vi "MRU_UpdateMRUList.vi"(8 "error in (no error)":errorcluster, 11 "reference in":refnum<class "MRU.lvclass">) -> (0 "error out":errorcluster, 3 "reference out":refnum<class "MRU.lvclass">)   [LabVIEW 2014, in "MRU.lvclass"]
doc: "Captures the current values in the Combo Box and saves them to the INI file given to the constructor."
uses:
  MRU.lvclass
  <vilib>/Utility/config.llb/Write Key (String).vi
  <vilib>/Utility/config.llb/NI_LVConfig.lvlib
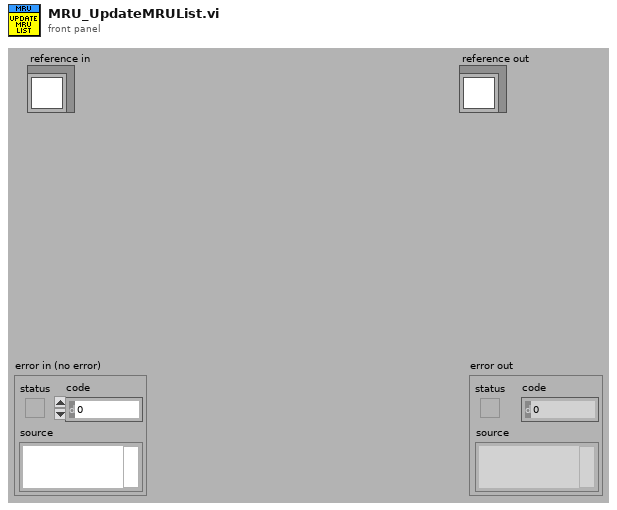
[diagram p1: front panel]
types:
  T1 = typedef "MRU.lvclass/ObjectAttributes.ctl" = cluster{"MRU INI file":path, "MRU Section Name":string, "CmbBox Refnum":refnum<vi>, "Number to remember":i32}
  T2 = typedef "NI_LVConfig.lvlib/Config Data RefNum.ctl" = refnum<k1>
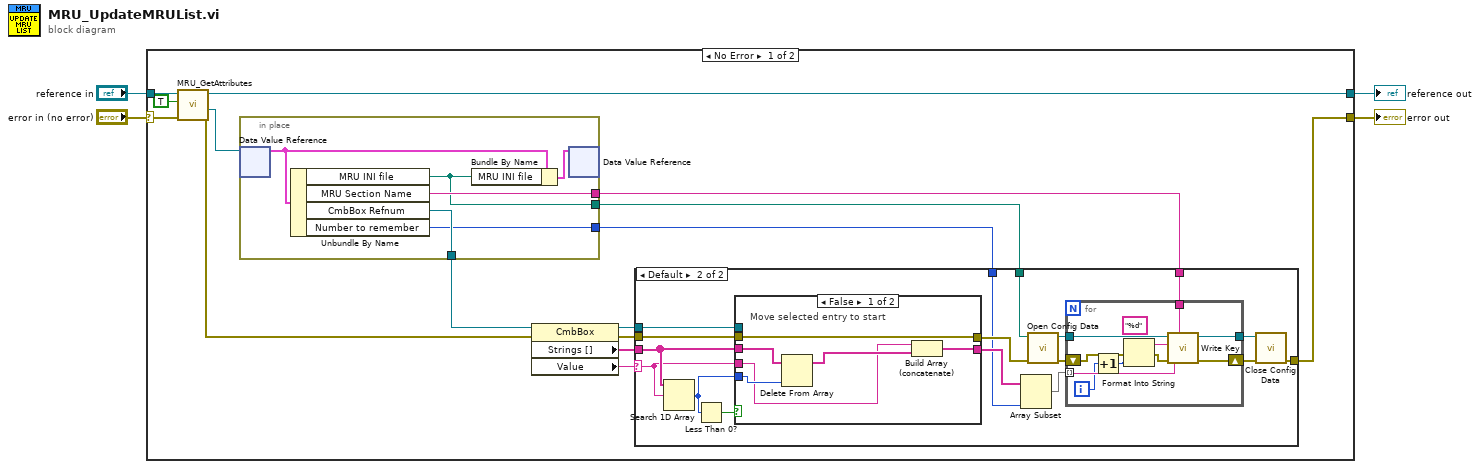
[diagram p0: block diagram]
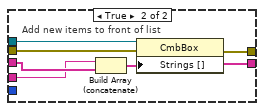
[diagram p3: hidden frame]
diagram:
  n1 = case shown="No Error" "error in (no error)" {
    selector: "error in (no error)" -> [w17 w68]
    tunnel: [w19 w68] -> w3
    tunnel: [w16 w67] -> w1
    tunnel: "reference in" -> [w18 w67]
    frame No Error {
      n2 = call "MRU_GetAttributes.vi"("error in (no error)"=w17, "OnlyGetDvrReference(False)"=TRUE, "reference in"=w18) -> ("error out"=w12:errorcluster, "DataRef"=w10:refnum<data-value>, "reference out"=w16:refnum<class "MRU.lvclass">)  [unwired: 5 in, 1 out]
      n3 = in-place {
        in-place-border: [w64] -> w9
        in-place-border: [w63] -> w8
        in-place-border: [w62] -> w7
        in-place-border: [w61] -> w6
        n4 = in-place-dvr #1(w10) -> (w66:T1)  [unwired: 1 out]
        n5 = Unbundle By Name(w66) -> ("MRU INI file"=w61:path, "MRU Section Name"=w64:string, "CmbBox Refnum"=w63:refnum<vi>, "Number to remember"=w62:i32)
        n6 = Bundle By Name(cluster=w66, "MRU INI file"=w61) -> (w65:T1)
        n7 = in-place-dvr #1(w65) -> ()  [unwired: 2 out]
      }
      n8 = property on="Property Node" class="CmbBox"(reference=w8, error in=w12) -> (reference out=w13:refnum<vi>, error out=w14:errorcluster, "Strings []"=w15:string[], "Value"=w5:string)
      n9 = case shown="Default" w5 {
        selector: w5 -> [_ w21]
        tunnel: [w20 w37] -> w19
        tunnel: w15 -> [_ w35]
        tunnel: w14 -> [w20 w34]
        tunnel: w13 -> [_ w28]
        tunnel: w9 -> [_ w24]
        tunnel: w7 -> [_ w23]
        tunnel: w6 -> [_ w22]
        frame "\u0000" {
        }
        frame Default {
          n10 = Search 1D Array(1D array=w35, element=w21) -> (index of element=w25:i32)  [unwired: 1 out]
          n11 = Less Than 0?(x=w25) -> (x < 0?=w36:bool)
          n12 = case shown="False" w36 {
            tunnel: w35 -> [w53 w56]
            tunnel: w21 -> [w50 w55]
            tunnel: [w49 w60] -> w26
            tunnel: w34 -> [w54 w59]
            tunnel: [w54 w58] -> w29
            tunnel: w28 -> [_ w57]
            tunnel: w25 -> [w52 _]
            frame False {
              # "Move selected entry to start"
              n13 = Delete From Array(array=w53, index=w52) -> (array with subset deleted=w51:string[])  [unwired: 1 in, 1 out]
              n14 = Build Array (concatenate)(w50, w51) -> (w49:string[])
            }
            frame True {
              # "Add new items to front of list"
              n15 = Build Array (concatenate)(w55, w56) -> (w60:string[])
              n16 = property on="Property Node" class="CmbBox"(reference=w57, error in=w59, "Strings []"=w60) -> (error out=w58:errorcluster)  [unwired: 1 out]
            }
          }
          n17 = Array Subset(array=w26, length=w23) -> (w27:string[])  [unwired: 1 in]
          n18 = call <vilib>:"Open Config Data.vi"("error in (no error)"=w29, "configuration file path"=w22) -> ("error out"=w33:errorcluster, "refnum"=w31:T2)  [unwired: 7 in, 1 out]
          n19 = for {
            tunnel: w31 -> [w47]
            tunnel: [w46] -> w30
            shift-right: [w48] -> w32
            shift-left: w33 -> [w42]
            tunnel: w24 -> [w45]
            tunnel: w27 -> [w40] mode=indexing
            i -> [w39]
            n20 = Increment(x=w39) -> (x+1=w38:i32)
            n21 = Format Into String(format string="%d", error in=w42, w38) -> (resulting string=w43:string, error out=w41:errorcluster)  [unwired: 1 in]
            n22 = call-poly <vilib>:"Write Key.vi"("section"=w45, "error in (no error)"=w41, "value"=w40, "key"=w43, "refnum"=w47) -> ("error out"=w48:errorcluster, "refnum out"=w46:T2)  [unwired: 1 in, 4 out]
          }
          n23 = call <vilib>:"Close Config Data.vi"("error in (no error)"=w32, "refnum"=w30) -> ("error out"=w37:errorcluster)  [unwired: 1 in, 8 out]
        }
      }
    }
    frame Error {
    }
  }
  "error out" <- w3
  "reference out" <- w1
